vi "process_signals.vi"(8 "error in (no error)":errorcluster, 11 "data":waveform(dbl)[](array[waveform])) -> (0 "SUM":waveform(dbl), 1 "MT":waveform(dbl)[](array[waveform]), 2 "BT":waveform(dbl), 3 "LR":waveform(dbl), 4 "error out":errorcluster)   [LabVIEW 2026]
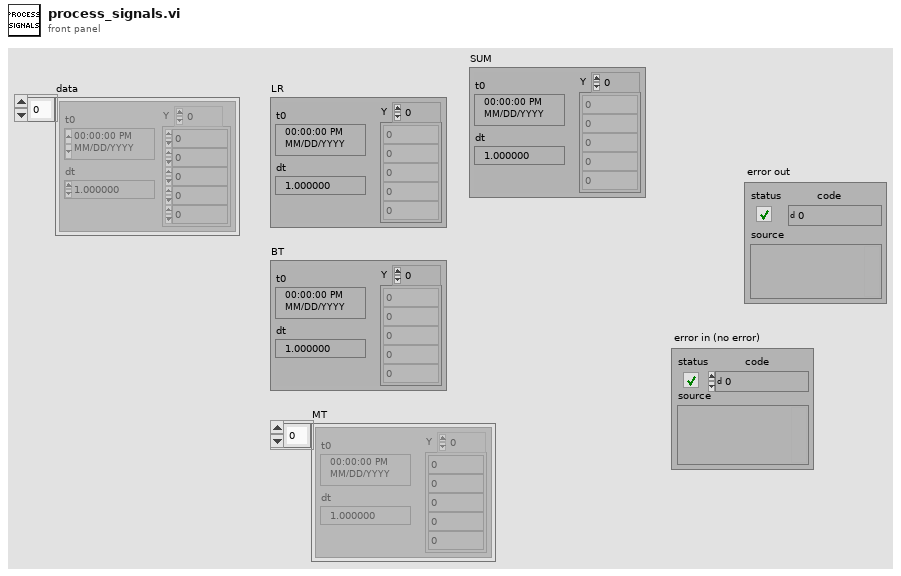
[diagram p1: front panel]
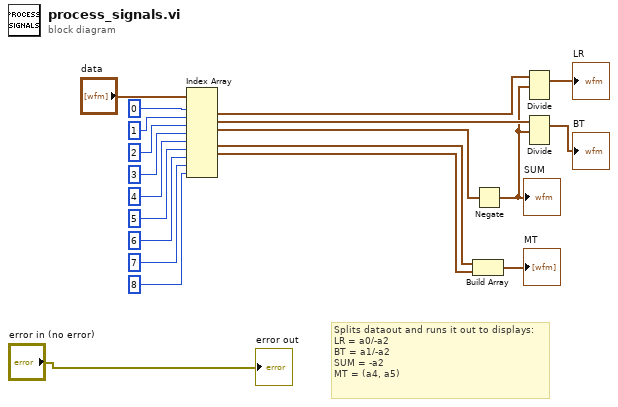
[diagram p0: block diagram]
diagram:
  # "Splits dataout and runs it out to displays:\nLR = a0/-a2\nBT = a1/-a2\nSUM = -a2\nMT = (a4, a5)"
  n1 = Index Array(array="data", index #1=0 ("index"), index #2=1 ("index"), index #3=2 ("index"), index #4=3 ("index"), index #5=4 ("index"), index #6=5 ("index"), index #7=6 ("index"), index #8=7 ("index"), index #9=8 ("index")) -> (element #1=w13:waveform(dbl), element #2=w14:waveform(dbl), element #3=w12:waveform(dbl), element #5=w17:waveform(dbl), element #6=w18:waveform(dbl))  [unwired: 4 out]
  n2 = Build Array(w17, w18) -> (→"MT":waveform(dbl)[])
  n3 = Negate(x=w12) -> (-x=w2:waveform(dbl))
  "SUM" <- w2
  n4 = Divide(1:w2, 2:w13) -> (0:→"LR":waveform(dbl))  [unwired: 1 in, 1 out]
  n5 = Divide(1:w2, 2:w14) -> (0:→"BT":waveform(dbl))  [unwired: 1 in, 1 out]
  "error out" <- "error in (no error)"
